vi "Get Config File Path.vi"(8 "error in (no error)":errorcluster, 10 "Settings File Name":string) -> (0 "error out":errorcluster, 3 "XML File Path":path)   [LabVIEW 2017, in "Settings.lvlib"]
doc: "Get the path to the Settings XML file. This is done using the Application Directory function. For more information on how Application Directory calculates its path, right-click the function and choose Help."
uses:
  Settings.lvlib
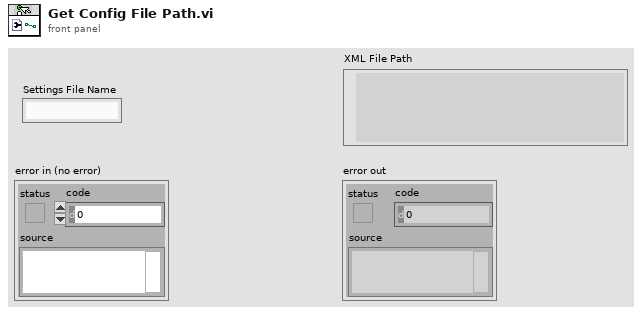
[diagram p1: front panel]
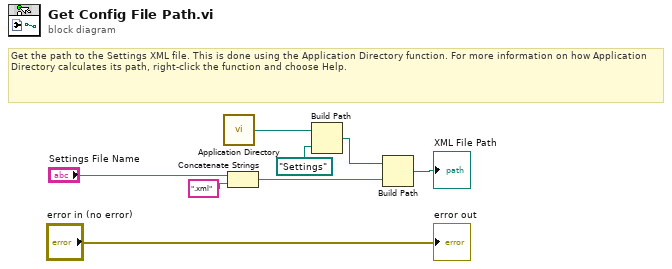
[diagram p0: block diagram]
diagram:
  # "Get the path to the Settings XML file. This is done using the Application Directory function. For more information on how Application Directory calculates its path, right-click the function and choose Help."
  n1 = call <vilib>:"Application Directory.vi"() -> ("Application Directory"=w3:path)
  n2 = Concatenate Strings("Settings File Name", ".xml" ("string")) -> (w6:string)
  n3 = Build Path(base path=w3, name or relative path=path "Settings" ("string")) -> (appended path=w4:path)
  n4 = Build Path(base path=w4, name or relative path=w6) -> (appended path=→"XML File Path":path)
  "error out" <- "error in (no error)"
